vi "aad2.vi"() -> ()   [LabVIEW 2024]
uses:
  <vilib>/Analysis/2dsp.llb/Real FFT.vi
  <vilib>/measure/maspectr.llb/FFT Spectrum (Mag-Phase) for 1 Chan.vi
  <vilib>/Analysis/NI_AALPro.lvlib
  <vilib>/measure/NI_MAPro.lvlib
panel:
  out "Mag-phase Graph":cluster{"f0":dbl, "df":dbl, "magnitude":dbl[]}(graph)
  out "Scale Graph":cluster{dbl, dbl, dbl[]}(graph)
  out "Array":dbl[](array[numeric])
  out "1/x":cluster{"X":dbl, "Y":dbl}
  out "FTT Graph":dbl[](graph)
  out "Data Graph":dbl[](graph)
  in  "stop":bool
  out "Read buffer":string="200\r\n268\r\n2BE\r\n2F3\r\n2FF\r\n2DE\r\n296\r\n235\r\n1CB\r\n16A\r\n122\r\n101\r\n10D\r\n142\r\n198\r\n200\r\n268\r\n2BE\r\n2F3\r\n2FF\r\n2DE\r\n296\r\n235\r\n1CB\r\n16A\r\n122\r\n101\r\n10D\r\n142\r\n198\r\n200\r\n268\r\n2BE\r\n2F3\r\n2FF\r\n2DE\r\n296\r\n235\r\n1CB\r\n16A\r\n122\r\n101\r\n10D\r\n142\r\n198\r\n200\r\n268\r\n2BE\r\n2F3\r\n2FF\r\n2DE\r\n296\r\n235\r\n1CB\r\n16A\r\n122\r\n101\r\n10D\r\n142\r\n198\r\n200\r\n268\r\n2BE\r\n2F3\r\n2FF\r\n2DE\r\n296\r\n235\r\n1CB\r\n16A\r\n122\r\n101\r\n10D\r\n142\r\n198\r\n200\r\n268\r\n2BE\r\n2F3\r\n2FF\r\n2DE\r\n296\r\n235\r\n1CB\r\n16A\r\n122\r\n101\r\n10D\r\n142\r\n198\r\n200\r\n268\r\n2BE\r\n2F3\r\n2FF\r\n2DE\r\n296\r\n235\r\n1CB\r\n16A\r\n122\r\n101\r\n10D\r\n142\r\n198\r\n200\r\n268\r\n2BE\r\n2F3\r\n2FF\r\n2DE\r\n296\r\n235\r\n1CB\r\n16A\r\n122\r\n101\r\n10D\r\n142\r\n198\r\n..."
  in  "Sine Wave":T1={"Frequency [Hz]"=50.0, "Amplitude [V]"=2.0, "Offset [V]"=2.5}
  in  "byte count":u32
  in  "RUN":bool
  # "dont forget to put bytes"
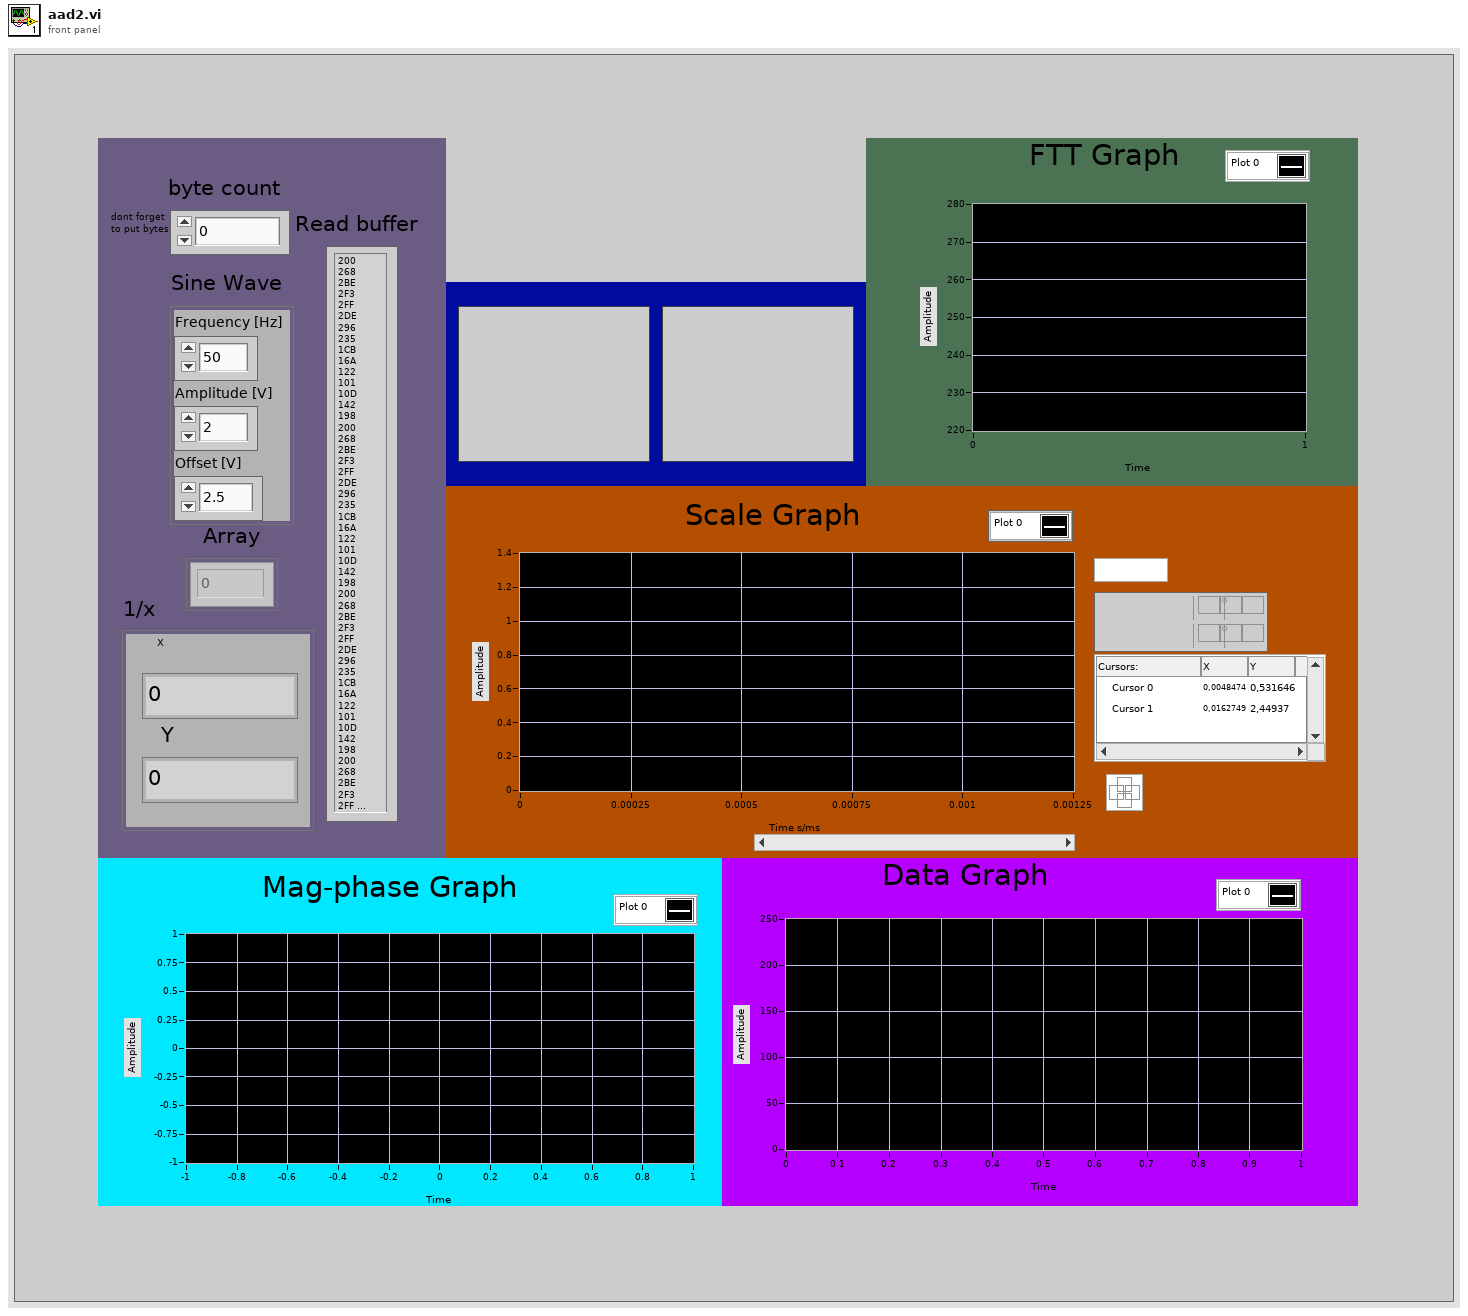
[diagram p1: front panel]
types:
  T1 = cluster{"Frequency [Hz]":dbl, "Amplitude [V]":dbl, "Offset [V]":dbl}
  T2 = typedef "LVCursorListTypeDef.ctl" = cluster{"Name":string, "Color":u32, "Style":u8, "Point Style":u8, "Name Visible":bool, "Allow Drag":bool, "Cursor Mode":u32, "Plot":i32, "Index":i32, "Position":cluster{"X":dbl, "Y":dbl}, "X Scale":u32, "Y Scale":u32, "Watch Plots":i32[], "Watch All Plots":bool, "Plot Area":i32, "Label Offset":cluster{"X":dbl, "Y":dbl}}[]
  T3 = cluster{"Name":string, "Color":u32, "Style":u8, "Point Style":u8, "Name Visible":bool, "Allow Drag":bool, "Cursor Mode":u32, "Plot":i32, "Index":i32, "Position":cluster{"X":dbl, "Y":dbl}, "X Scale":u32, "Y Scale":u32, "Watch Plots":i32[], "Watch All Plots":bool, "Plot Area":i32, "Label Offset":cluster{"X":dbl, "Y":dbl}}
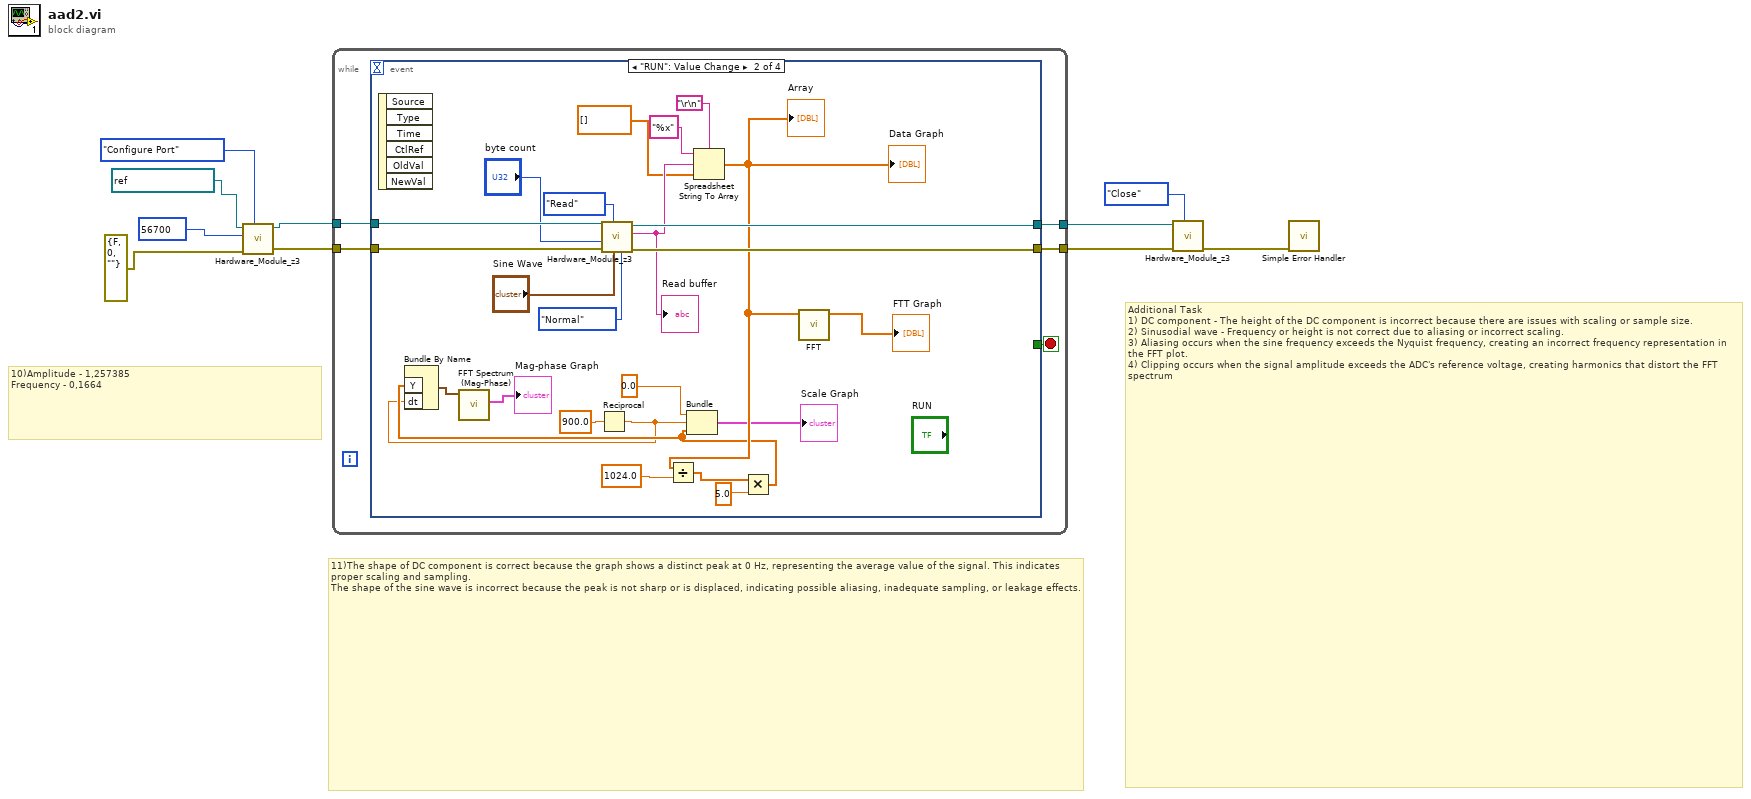
[diagram p0: block diagram]
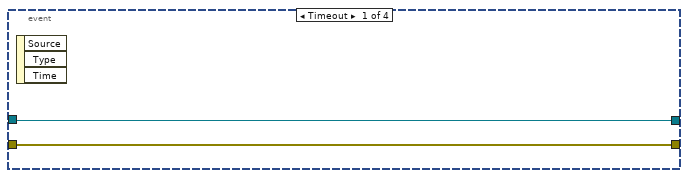
[diagram p2: hidden frame]
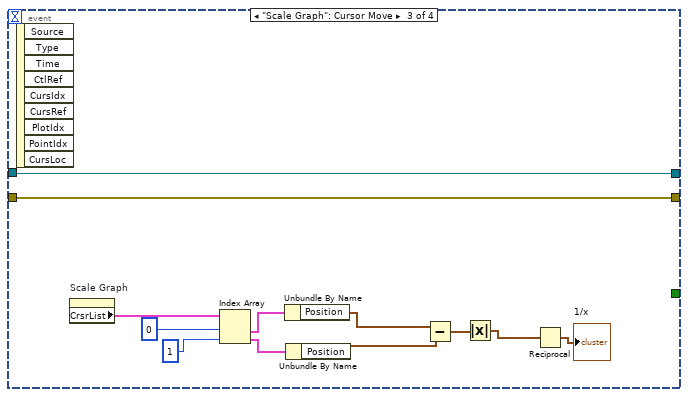
[diagram p3: hidden frame]
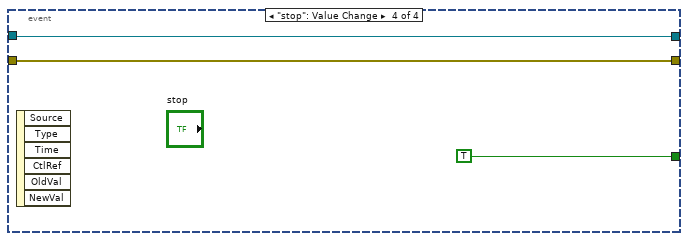
[diagram p4: hidden frame]
diagram:
  # "Additional Task\n1) DC component - The height of the DC component is incorrect because there are issues with scaling or sample size.\n2) Sinusodial wave - Frequency or height is not correct due to aliasing or incorrect scaling.\n3) Aliasing occurs when the sine frequency exceeds the Nyquist frequency, creating an incorrect frequency representation in the FFT plot.\n4) Clipping occurs when the signal amplitude exceeds the ADC's reference voltage, creating harmonics that distort the FFT spectrum"
  # "11)The shape of DC component is correct because the graph shows a distinct peak at 0 Hz, representing the average value of the signal. This indicates proper scaling and sampling.\nThe shape of the sine wave is incorrect because the peak is not sharp or is displaced, indicating possible aliasing, inadequate sampling, or leakage effects."
  # "10)Amplitude - 1,257385\nFrequency - 0,1664"
  n1 = call "Hardware_Module_z3.vi"("State"=enum16{"Configure Port", "Read", "Close"}."Configure Port", "error in (no error)"=errorcluster {"status"=FALSE, "code"=0, "source"=""} ("error constant"), "baud rate (9600)"=u32 56700, "VISA resource name"=refnum<visa-resource-name> "VirtualDevice1") -> ("error out"=w5:errorcluster, "VISA resource name out"=w6:refnum<visa-resource-name>)  [unwired: 5 in, 1 out]
  n2 = while {
    tunnel: w6 -> [w15]
    tunnel: w5 -> [w14]
    tunnel: [w13] -> w4
    tunnel: [w12] -> w3
    stop <- w11 stop-if-true
    n3 = event shown="[1] \"RUN\": Value Change" {
      selector: _ -> [_ _ _ _]
      dyn-events: _ -> [_ _ _ _]
      timeout: _ -> [_ _ _ _]
      tunnel: w15 -> [w17 w41 w45 w55]
      tunnel: w14 -> [w16 w40 w44 w54]
      tunnel: [w17 w36 w45 w55] -> w13
      tunnel: [w16 w35 w44 w54] -> w12
      tunnel: [_ _ _ TRUE] -> w11
      event Timeout {
        n4 = event-data() -> ()  [unwired: 1 in, 3 out]
      }
      event "RUN": Value Change {
        n5 = event-data() -> ()  [unwired: 1 in, 6 out]
        n6 = Reciprocal(x=900.0) -> (1/x=w19:dbl)
        n7 = call "Hardware_Module_z3.vi"("Mode"=enum16{"Normal", "Hidden"}."Normal", "Sine Wave"="Sine Wave", "State"=enum16{"Configure Port", "Read", "Close"}."Read", "error in (no error)"=w40, "byte count"="byte count", "VISA resource name"=w41) -> ("error out"=w35:errorcluster, "read buffer"=w32:string, "VISA resource name out"=w36:refnum<visa-resource-name>)  [unwired: 3 in]
        "Read buffer" <- w32
        n8 = Spreadsheet String To Array(delimiter (Tab)="\r\n", format string="%x", spreadsheet string=w32, array type (2D Dbl)=dbl[] []) -> (array=w27:dbl[])
        "Data Graph" <- w27
        "Array" <- w27
        n9 = Divide(x=w27, y=1024.0) -> (x/y=w25:dbl[])
        n10 = Multiply(x=w25, y=5.0) -> (x*y=w21:dbl[])
        n11 = Bundle By Name("Y"=w21, "dt"=w19) -> (w22:waveform(dbl))  [unwired: 1 in]
        n12 = call-poly <vilib>:"FFT Spectrum (Mag-Phase).vi"("time signal"=w22) -> ("phase"=→"Mag-phase Graph":cluster{"f0":dbl, "df":dbl, "phase":dbl[]})  [unwired: 6 in, 4 out]
        n13 = Bundle(0.0, w19, w21) -> (→"Scale Graph":cluster{dbl, dbl, dbl[]})  [unwired: 1 in]
        n14 = call-poly <vilib>:"FFT.vi"("X"=w27) -> ("FFT {X}"=→"FTT Graph":cdb[])  [unwired: 9 in, 1 out]
      }
      event "Scale Graph": Cursor Move {
        n15 = event-data() -> ()  [unwired: 1 in, 9 out]
        n16 = property on="Scale Graph" class="WFGraph (strict)"() -> ("CrsrList"=w46:T2)  [unwired: 2 in, 2 out]
        n17 = Index Array(array=w46, index #1=0 ("index"), index #2=1 ("index")) -> (element #1=w53:T3, element #2=w52:T3)
        n18 = Unbundle By Name(w53) -> ("Position"=w51:cluster{"X":dbl, "Y":dbl})
        n19 = Unbundle By Name(w52) -> ("Position"=w43:cluster{"X":dbl, "Y":dbl})
        n20 = Subtract(x=w51, y=w43) -> (x-y=w48:cluster{"X":dbl, "Y":dbl})
        n21 = Absolute Value(x=w48) -> (abs(x)=w47:cluster{"X":dbl, "Y":dbl})
        n22 = Reciprocal(x=w47) -> (1/x=→"1/x":cluster{"X":dbl, "Y":dbl})
      }
      event "stop": Value Change {
        n23 = event-data() -> ()  [unwired: 1 in, 6 out]
      }
    }
  }
  n24 = call "Hardware_Module_z3.vi"("State"=enum16{"Configure Port", "Read", "Close"}."Close", "error in (no error)"=w3, "VISA resource name"=w4) -> ("error out"=w1:errorcluster)  [unwired: 6 in, 2 out]
  n25 = call <vilib>:"Simple Error Handler.vi"("error in (no error)"=w1) -> ()  [unwired: 4 in, 5 out]
